vi "Simple Reader.vi"(8 "error in (no error)":errorcluster, 11 "Arduino Temperature Controller Driver in":refnum<class "Arduino Temperature Controller Driver.lvclass">) -> (0 "error out":errorcluster, 2 "Signals":dbl[](array[numeric]), 3 "Arduino Temperature Controller Driver out":refnum<class "Arduino Temperature Controller Driver.lvclass">)   [LabVIEW 2019, in "Arduino Temperature Controller Driver.lvclass"]
uses:
  Arduino Temperature Controller Driver.lvclass
  C:/GitHub/NHMFL_Core/Libraries/Instruments/VISA Instrument/VISA Instrument.lvclass
  C:/GitHub/NHMFL_Core/Libraries/Instruments/Temperature Controller Driver/Temperature Controller Driver.lvclass
  VISA Instrument/VISA Instrument.lvclass/VISA Instrument.ctl
  VISA Instrument/Read VISA resource.vi
  VISA Instrument/Write VISA resource.vi
  Temperature Controller Driver/Read T controller configuration.vi
panel:
  out "Array - String":string[](array[string])
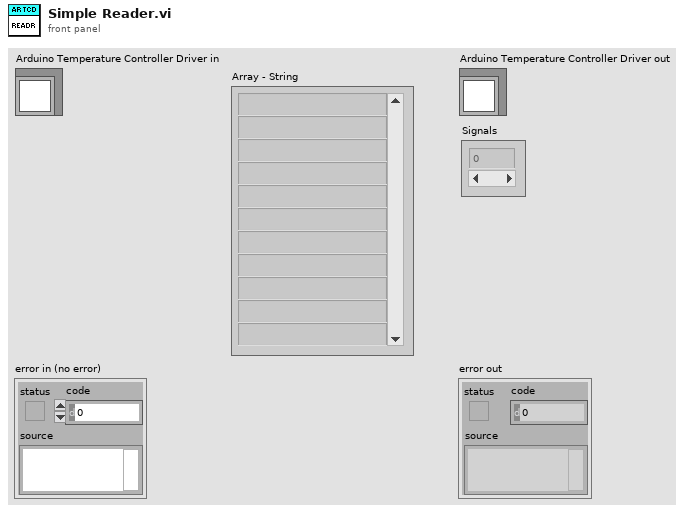
[diagram p1: front panel]
types:
  T1 = typedef "T controller configuration.ctl" = cluster{"Record Channels":string[], "Add raw signal":bool, "New set point":dbl, "Record heater":bool}
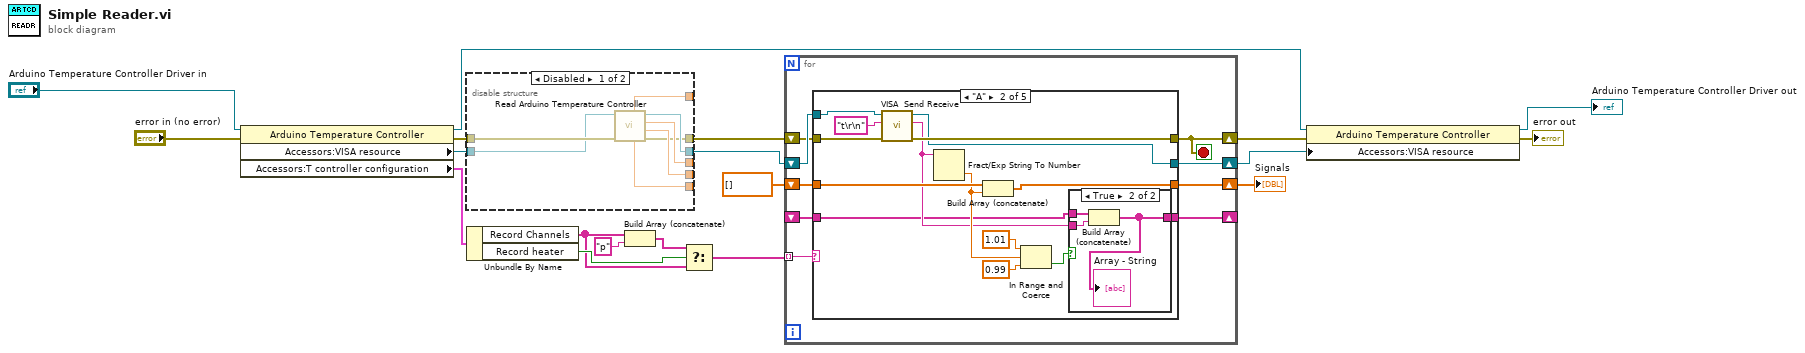
[diagram p0: block diagram]
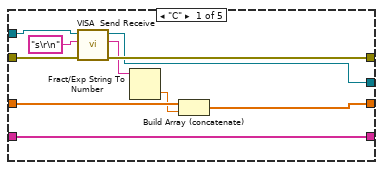
[diagram p3: hidden frame]
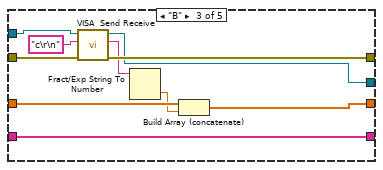
[diagram p5: hidden frame]
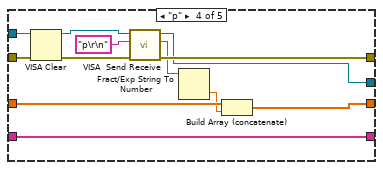
[diagram p6: hidden frame]
diagram:
  n1 = property class="Arduino Temperature Controller "(reference="Arduino Temperature Controller Driver in", error in="error in (no error)") -> (reference out=w18:refnum<class "Arduino Temperature Controller Driver.lvclass">, error out=w13:errorcluster, "Accessors:VISA resource"=w4:refnum<visa-resource-name>, "Accessors:T controller configuration"=w19:T1)
  n2 = disable-structure shown="Disabled" {
    disable-tunnel: w13 -> [w27 w28]
    disable-tunnel: [w26 w29] -> w3
    disable-tunnel: [w25 _] -> _
    disable-tunnel: [w24 _] -> _
    disable-tunnel: [w23 _] -> _
    disable-tunnel: [w22 _] -> _
    disable-tunnel: w4 -> [w21 w29]
    disable-tunnel: [w20 w28] -> w10
    frame Disabled {
      n3 = call "Read Arduino Temperature Controller.vi"("Error In"=w27, "VISA resource name"=w21) -> ("Error Out"=w20:errorcluster, "Control temperature"=w24:dbl, "Sample temperature"=w25:dbl, "VISA resource name out"=w26:refnum<visa-resource-name>, "Power"=w23:dbl, "Set point"=w22:dbl)  [unwired: 4 in]
    }
    frame Enabled {
    }
  }
  n4 = Unbundle By Name(w19) -> ("Record Channels"=w6:string[], "Record heater"=w9:bool)
  n5 = Build Array (concatenate)(w6, "p") -> (w7:string[])
  n6 = Select(t=w7, s=w9, f=w6) -> (s? t:f=w5:string[])
  n7 = for {
    tunnel: w5 -> [w38] mode=indexing
    shift-right: [w32] -> w11
    shift-left: dbl[] [] -> [w33]
    shift-right: [w34] -> w2
    shift-left: w3 -> [w37]
    shift-right: [w35] -> w1
    shift-left: w10 -> [w36]
    shift-right: [w31] -> _
    shift-left: _ -> [w30]
    stop <- w35 stop-if-true
    n8 = case shown="\"A\"" w38 {
      tunnel: w37 -> [w48 w62 w76 w88 w92]
      tunnel: w36 -> [w47 w61 w75 w79 w91]
      tunnel: [w46 w60 w74 w87 w91] -> w35
      tunnel: [w45 w59 w73 w86 w92] -> w34
      tunnel: w33 -> [w44 w58 w72 w85 w90]
      tunnel: [w43 w57 w71 w84 w90] -> w32
      tunnel: [w39 w50 w67 w77 w89] -> w31
      tunnel: w30 -> [w39 w49 w67 w77 w89]
      frame "C" {
        n9 = call "VISA  Send Receive.vi"("error in (no error)"=w47, "data string in"="s\r\n" ("write buffer"), "VISA Resource Name"=w48) -> ("error out"=w46:errorcluster, "data string out"=w42:string, "VISA Resource Name Out"=w45:refnum<visa-resource-name>)  [unwired: 6 in]
        n10 = Fract/Exp String To Number(string=w42) -> (number=w41:dbl)  [unwired: 3 in, 1 out]
        n11 = Build Array (concatenate)(w44, w41) -> (w43:dbl[])
      }
      frame "A" {
        n12 = call "VISA  Send Receive.vi"("error in (no error)"=w61, "data string in"="t\r\n" ("write buffer"), "VISA Resource Name"=w62) -> ("error out"=w60:errorcluster, "data string out"=w51:string, "VISA Resource Name Out"=w59:refnum<visa-resource-name>)  [unwired: 6 in]
        n13 = Fract/Exp String To Number(string=w51) -> (number=w55:dbl)  [unwired: 3 in, 1 out]
        n14 = Build Array (concatenate)(w58, w55) -> (w57:dbl[])
        n15 = In Range and Coerce(upper limit=1.01, x=w55, lower limit=0.99) -> (In Range?=w52:bool)  [unwired: 1 out]
        n16 = case shown="True" w52 {
          tunnel: w51 -> [_ w66]
          tunnel: [w63 w64] -> w50
          tunnel: w49 -> [w63 w65]
          frame False {
          }
          frame True {
            n17 = Build Array (concatenate)(w65, w66) -> (w64:string[])
            "Array - String" <- w64
          }
        }
      }
      frame "B" {
        n18 = call "VISA  Send Receive.vi"("error in (no error)"=w75, "data string in"="c\r\n" ("write buffer"), "VISA Resource Name"=w76) -> ("error out"=w74:errorcluster, "data string out"=w70:string, "VISA Resource Name Out"=w73:refnum<visa-resource-name>)  [unwired: 6 in]
        n19 = Fract/Exp String To Number(string=w70) -> (number=w69:dbl)  [unwired: 3 in, 1 out]
        n20 = Build Array (concatenate)(w72, w69) -> (w71:dbl[])
      }
      frame "p" {
        n21 = VISA Clear(VISA resource name=w88, error in (no error)=w79) -> (VISA resource name out=w80:refnum<visa-resource-name>, error out=w78:errorcluster)
        n22 = call "VISA  Send Receive.vi"("error in (no error)"=w78, "data string in"="p\r\n" ("write buffer"), "VISA Resource Name"=w80) -> ("error out"=w87:errorcluster, "data string out"=w83:string, "VISA Resource Name Out"=w86:refnum<visa-resource-name>)  [unwired: 6 in]
        n23 = Fract/Exp String To Number(string=w83) -> (number=w82:dbl)  [unwired: 3 in, 1 out]
        n24 = Build Array (concatenate)(w85, w82) -> (w84:dbl[])
      }
      frame "", Default {
      }
    }
  }
  "Signals" <- w11
  n25 = property class="Arduino Temperature Controller "(reference=w18, error in=w1, "Accessors:VISA resource"=w2) -> (reference out=→"Arduino Temperature Controller Driver out":refnum<class "Arduino Temperature Controller Driver.lvclass">, error out=→"error out":errorcluster)
